vi "MasterRobotModeController.vi"() -> (1 "FMS Robot Mode":T1, 2 "Auto Reset":bool, 3 "Robot is Autonomous":bool)   [LabVIEW 2023]
doc: "This state controller manages the Robot Mode and whether or not the robot is running autonomously. The robot will continue running autonomously after Autonomous Mode ends, until the driver touches the joystick during TeleOperated Mode or until/unless the FORCE HUMAN CONTROL override is flipped on the FRC 4265 Dashboard."
uses:
  <vilib>/Rock Robotics/WPI/DriverStation/WPI_DriverStationRobotMode2.ctl
  GlobalDriverStationData.vi
  GlobalDriverStationCommands.vi
  GRNF_Joystick.vi
  GlobalAutonomous.vi
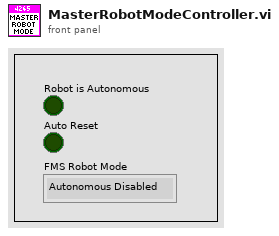
[diagram p1: front panel]
types:
  T1 = typedef "WPI_DriverStationRobotMode2.ctl" = enum16{"Autonomous Disabled", "Autonomous Enabled", "Teleop Disabled", "Teleop Enabled", "Disconnected", "Finish", "Test Disabled", "Test Enabled", "Emergency Stopped"}
  T2 = typedef "WPI_JoystickDevRef.ctl" = cluster{"Device":T3}
  T3 = typedef "WPI_JoystickDeviceEnum.ctl" = enum16{"USB 0", "USB 1", "USB 2", "USB 3", "USB 4", "USB 5"}
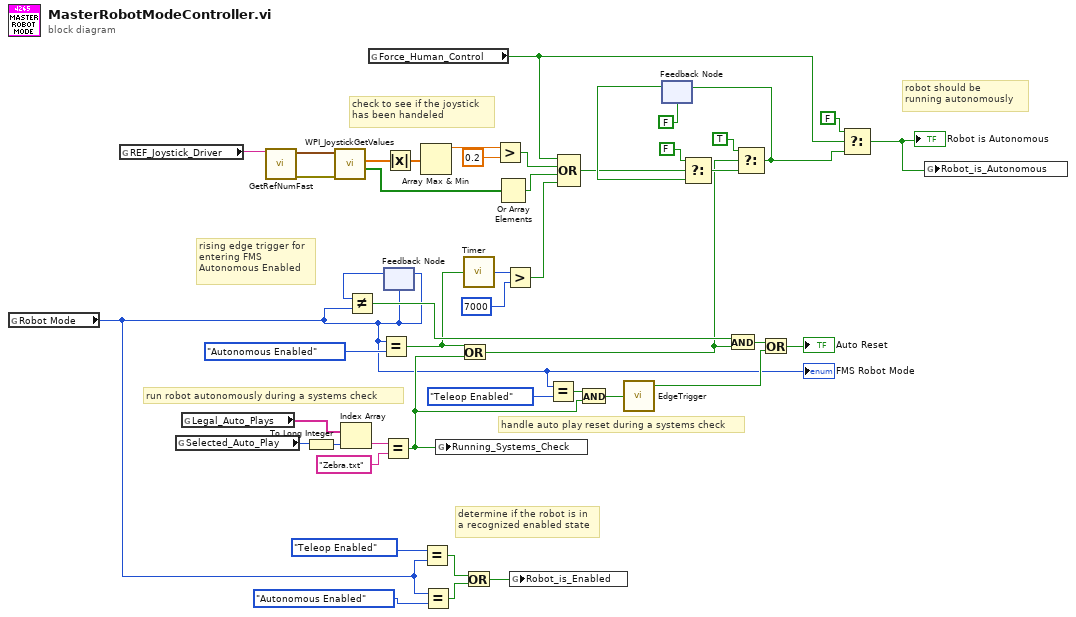
[diagram p0: block diagram]
diagram:
  # "determine if the robot is in\na recognized enabled state"
  # "handle auto play reset during a systems check"
  # "run robot autonomously during a systems check"
  # "rising edge trigger for\nentering FMS\nAutonomous Enabled"
  # "robot should be\nrunning autonomously"
  # "check to see if the joystick \nhas been handeled"
  n1 = global read "GlobalDriverStationData.vi" "Robot Mode"() -> (w4:T1)
  "FMS Robot Mode" <- w4
  n2 = global read "GlobalDriverStationCommands.vi" "REF_Joystick_Driver"() -> (w8:string)
  n3 = global read "GlobalDriverStationData.vi" "Selected_Auto_Play"() -> (w20:u16)
  n4 = global read "GlobalAutonomous.vi" "Legal_Auto_Plays"() -> (w7:string[])
  n5 = call-poly "GetRefNumFast.vi"("RefNum Name"=w8) -> ("Error"=w45:errorcluster, "Device Reference"=w46:T2)  [unwired: 5 in]
  n6 = To Long Integer(number=w20) -> (32bit integer=w21:i32)
  n7 = call <vilib>:"WPI_JoystickGetValues.vi"("error in (no error)"=w45, "JoystickDevRef"=w46) -> ("Buttons"=w44:bool[], "Axes"=w43:dbl[])  [unwired: 5 in, 3 out]
  n8 = Index Array(array=w7, index=w21) -> (element=w19:string)
  n9 = global read "GlobalDriverStationData.vi" "Force_Human_Control"() -> (w25:bool)
  n10 = Equal?(x=w4, y=WPI_DriverStationRobotMode2."Autonomous Enabled" ("Robot Mode")) -> (x = y?=w16:bool)
  n11 = Equal?(x=w19, y="Zebra.txt") -> (x = y?=w11:bool)
  n12 = feedback #1(w4) -> (w34:T1)
  n13 = Not Equal?(x=w34, y=w4) -> (x != y?=w33:bool)
  n14 = feedback-in #1(w4) -> ()
  n15 = Absolute Value(x=w43) -> (abs(x)=w42:dbl[])
  n16 = Array Max & Min(array=w42) -> (max value=w41:dbl)  [unwired: 3 out]
  n17 = Equal?(x=WPI_DriverStationRobotMode2."Teleop Enabled" ("Robot Mode"), y=w4) -> (x = y?=w3:bool)
  n18 = Equal?(x=w4, y=WPI_DriverStationRobotMode2."Autonomous Enabled" ("Robot Mode")) -> (x = y?=w2:bool)
  n19 = global write "GlobalDriverStationData.vi" "Running_Systems_Check"(w11) -> ()
  n20 = Or(x=w16, y=w11) -> (x .or. y?=w17:bool)
  n21 = call "Timer.vi"("Reset Timer"=w16) -> ("Time (ms)"=w24:u32)
  n22 = Or(x=w3, y=w2) -> (x .or. y?=w1:bool)
  n23 = Greater?(x=w41, y=0.2) -> (0:w39:bool)
  n24 = Or Array Elements(Boolean array=w44) -> (logical OR=w38:bool)
  n25 = Greater?(x=w24, y=u32 7000) -> (0:w22:bool)
  n26 = global write "GlobalDriverStationData.vi" "Robot_is_Enabled"(w1) -> ()
  n27 = Equal?(x=w4, y=WPI_DriverStationRobotMode2."Teleop Enabled" ("Robot Mode")) -> (x = y?=w12:bool)
  n28 = Compound Arithmetic op=OR(w25, w39, w38, w22) -> (w29:bool)
  n29 = And(x=w12, y=w11) -> (x .and. y?=w10:bool)
  n30 = call "EdgeTrigger.vi"("Input Signal"=w10) -> ("Rising Edge Trigger"=w9:bool)  [unwired: 2 out]
  n31 = feedback #2(FALSE) -> (w30:bool)
  n32 = Select(t=FALSE, s=w29, f=w30) -> (s? t:f=w31:bool)
  n33 = And(x=w33, y=w17) -> (x .and. y?=w15:bool)
  n34 = Select(t=TRUE, s=w17, f=w31) -> (s? t:f=w27:bool)
  n35 = feedback-in #2(w27) -> ()
  n36 = Or(x=w15, y=w9) -> (x .or. y?=→"Auto Reset":bool)
  n37 = Select(t=FALSE, s=w25, f=w27) -> (s? t:f=w26:bool)
  "Robot is Autonomous" <- w26
  n38 = global write "GlobalDriverStationData.vi" "Robot_is_Autonomous"(w26) -> ()
